vi "Not Equivalent.vi"(8 "Other JSON":string="{}", 10 "JSON":string="{}") -> (2 "Not Equivalent":bool caption="Not Equivalent (or invalid)")   [LabVIEW 2021, in "jsontext.facade.lvlib"]
doc: "Returns True if two JSON Values are \"Not Equivalent\".\n\nEqual means they are the same JSON infomation. Not considered differences are:\n -- different order of JSON Object items\n -- presence of any formating whitespace (outside of a JSON String)\n -- different formating of numbers (123.00 verus 123 or 1.23E2)\n\nNote: If using the LabVIEW extension that uses NaN numbers, these are considered Equivalent, ignoring the ususal convention of NaN not equal to NaN.\n\nInvalid JSON will always return \"Not Equivalent\" even if both inputs are identical.\n\nThis function looks only at the leading JSON Value in the input strings, ignoring any following characters."
uses:
  jsontext.facade.lvlib
  jsontext/JSONtext.lvlib
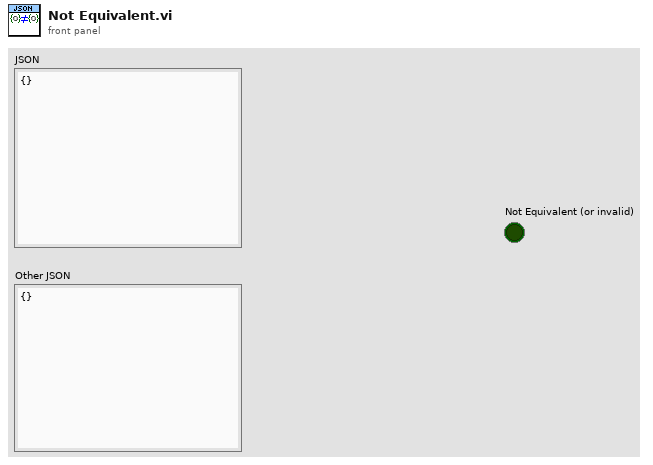
[diagram p1: front panel]
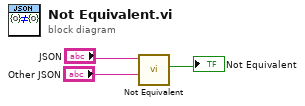
[diagram p0: block diagram]
diagram:
  n1 = call "Not Equivalent.vi"("Other JSON"="Other JSON", "JSON"="JSON") -> ("Not Equivalent"=→"Not Equivalent":bool)  [unwired: 8 in]
